vi "SDCP SMF Receiver and Transmitter - Generate Trace Info File.vi"(7 "Trace File Path":path, 8 "error in (no error)":errorcluster, 9 "Number of samples":u32, 10 "Stop Time":timestamp, 11 "Start Time":timestamp) -> (0 "error out":errorcluster)   [LabVIEW 2020]
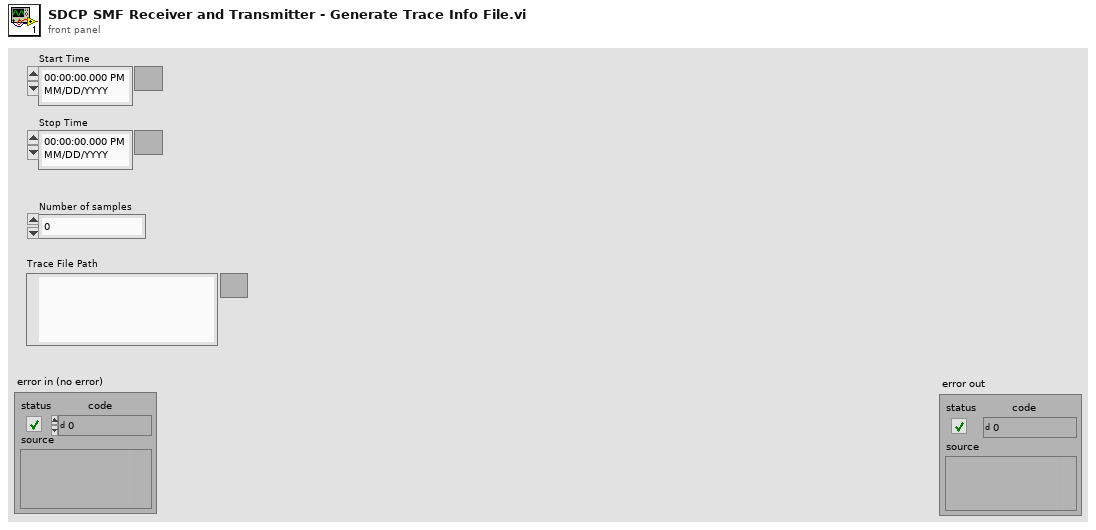
[diagram p1: front panel]
types:
  T1 = enum16{"open", "replace", "create", "open or create", "replace or create", "replace or create with confirmation"}
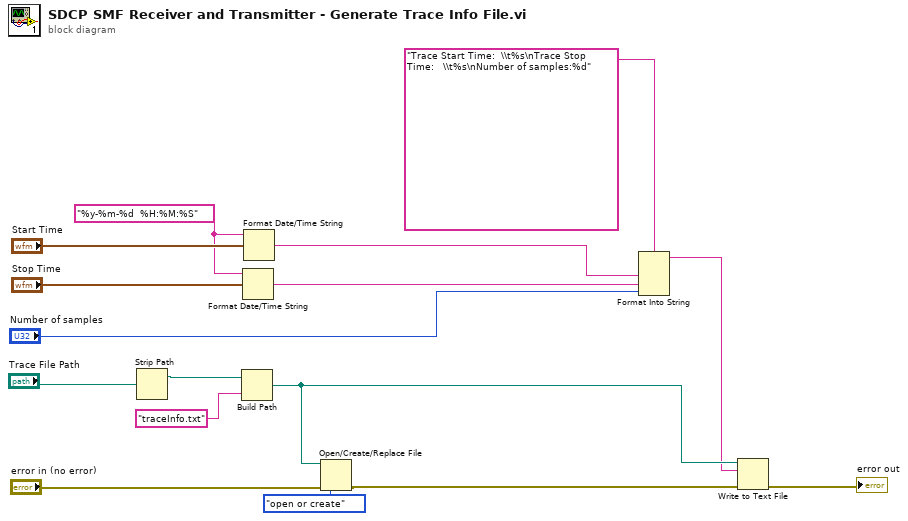
[diagram p0: block diagram]
diagram:
  w14 = "%y-%m-%d  %H:%M:%S" ("time format string (%c)")
  n1 = Strip Path(path="Trace File Path") -> (stripped path=w12:path)  [unwired: 1 out]
  n2 = Build Path(base path=w12, name or relative path="traceInfo.txt") -> (appended path=w3:path)
  n3 = Format Date/Time String(time format string (%c)=w14, seconds (now)="Stop Time") -> (date/time string=w6:string)  [unwired: 1 in]
  n4 = Format Date/Time String(time format string (%c)=w14, seconds (now)="Start Time") -> (date/time string=w7:string)  [unwired: 1 in]
  n5 = Open/Create/Replace File(file path (use dialog)=w3, error in="error in (no error)", operation (0:open)=T1."open or create") -> (error out=w4:errorcluster)  [unwired: 3 in, 2 out]
  n6 = Format Into String(format string="Trace Start Time:  \\t%s\nTrace Stop Time:   \\t%s\nNumber of samples:%d", w7, w6, "Number of samples") -> (resulting string=w2:string)  [unwired: 2 in, 1 out]
  n7 = Write to Text File(file (use dialog)=w3, text=w2, error in=w4) -> (error out=→"error out":errorcluster)  [unwired: 1 in, 2 out]
